vi "AC_OpenDriver.vi"() -> (0 "hDevice":u32 format="%x")   [LabVIEW 2015]
uses:
  acpci.dll
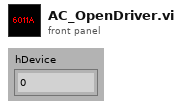
[diagram p1: front panel]
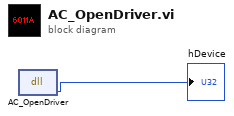
[diagram p0: block diagram]
diagram:
  n1 = dll-call lib="PTH2|abs F2.技术库labviewVI小程序:基于Labview的直流伺服电机位置控制系统设计\t源程序\tACPCI.DLL" fn="AC_OpenDriver"() -> (→"hDevice":u32)  [unwired: 3 in, 2 out]
